vi "String to temperature device cluster.vi"(11 "Temp Device Details":string="EXCT:TYPE:UNIP:MAG:0:STAT:40000000:NICK:MB1.T1:LOOP:AUX:None:D:1.0:HTR:None:I:1.0:THTF:None:HSET:0:PIDT:OFF:ENAB:OFF:SWFL:None:FAUT:OFF:FSET:0:PIDF:None:P:1.0:SWMD:FIX:TSET:0.0000K:MAN:HVER:1:FVER:1.12:SERL:111450078:CAL:OFFS:0:COLDL:999.00K:INT:LIN:SCAL:1:FILE:None:HOTL:999.00K:TYPE:TCE:SIG:VOLT:-0.0038mV:CURR:-0.0000A:TEMP:0.0000K:POWR:0.0000W:RES:0.0000O:SLOP:0.0000O/K") -> (3 "Temperature Device Settings":T1)   [LabVIEW 2014, in "Mercury iXX.lvlib" / "Temperature.lvlib"]
uses:
  Temperature.lvlib
  Controls/Temperature Device (Read).ctl
  Controls/Manufacturing Data.ctl
  Controls/Temperature Sensor Type.ctl
  Controls/Excitation Cluster.ctl
  Controls/Excitation Type.ctl
  Controls/Calibration Cluster.ctl
  Controls/Calibration Interpolation.ctl
  Controls/Loop Cluster.ctl
  Controls/Temperature Signals Cluster.ctl
  Mercury iXX.lvlib
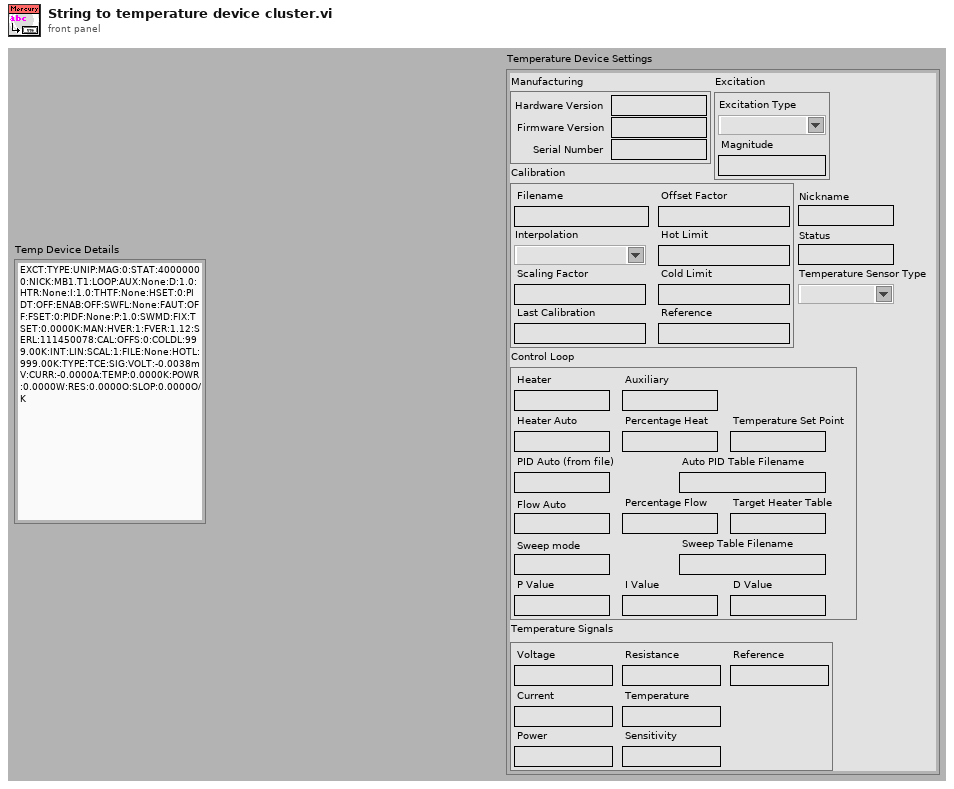
[diagram p1: front panel]
types:
  T1 = typedef "Mercury iXX.lvlib/Temperature.lvlib/Temperature Device (Read).ctl" = cluster{"Manufacturing":T2, "Temperature Sensor Type":T3, "Excitation":T4, "Calibration":T6, "Control Loop":T8, "Temperature Signals":T9, "Nickname":string, "Status":string}
  T2 = typedef "Mercury iXX.lvlib/Manufacturing Data.ctl" = cluster{"Hardware Version":string, "Firmware Version":string, "Serial Number":string}
  T3 = typedef "Mercury iXX.lvlib/Temperature.lvlib/Temperature Sensor Type.ctl" = string
  T4 = typedef "Mercury iXX.lvlib/Temperature.lvlib/Excitation Cluster.ctl" = cluster{"Excitation Type":T5, "Magnitude":string}
  T5 = typedef "Mercury iXX.lvlib/Temperature.lvlib/Excitation Type.ctl" = string
  T6 = typedef "Mercury iXX.lvlib/Temperature.lvlib/Calibration Cluster.ctl" = cluster{"Filename":string, "Interpolation":T7, "Scaling Factor":string, "Offset Factor":string, "Hot Limit":string, "Cold Limit":string, "Last Calibration":string, "Reference":string}
  T7 = typedef "Mercury iXX.lvlib/Temperature.lvlib/Calibration Interpolation.ctl" = string
  T8 = typedef "Mercury iXX.lvlib/Temperature.lvlib/Loop Cluster.ctl" = cluster{"Heater":string, "Auxiliary":string, "Heater Auto":string, "Percentage Heat":string, "Temperature Set Point":string, "PID Auto (from file)":string, "P Value":string, "I Value":string, "D Value":string, "Auto PID Table Filename":string, "Flow Auto":string, "Target Heater Table":string, "Sweep mode":string, "Sweep Table Filename":string, "Percentage Flow":string}
  T9 = typedef "Mercury iXX.lvlib/Temperature.lvlib/Temperature Signals Cluster.ctl" = cluster{"Voltage":string, "Current":string, "Power":string, "Resistance":string, "Temperature":string, "Sensitivity":string, "Reference":string}
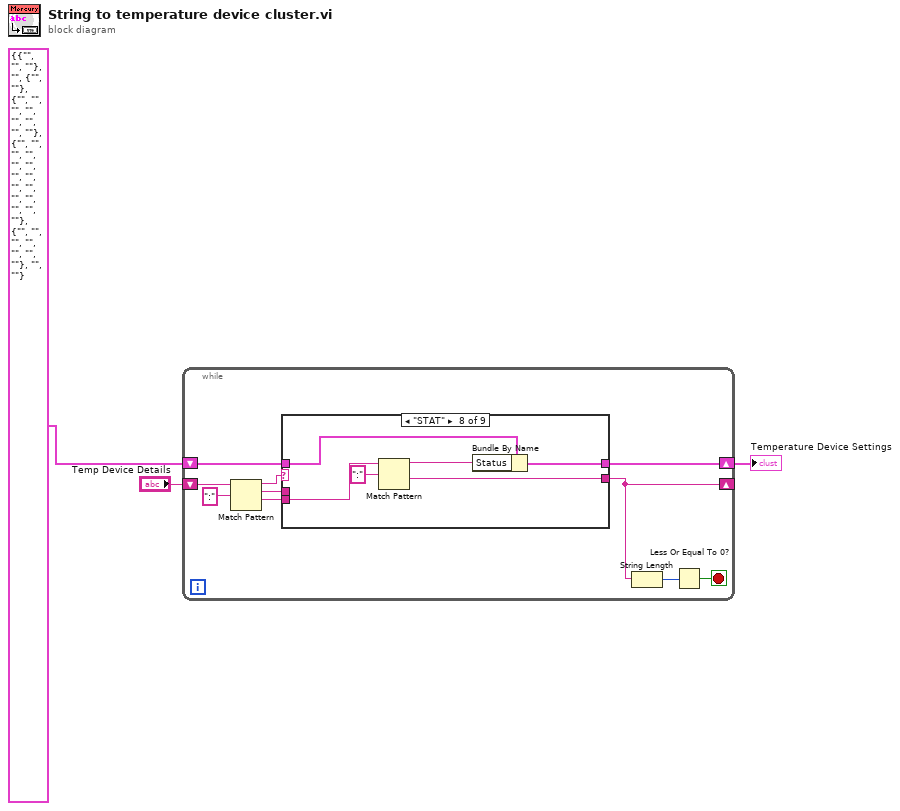
[diagram p0: block diagram]
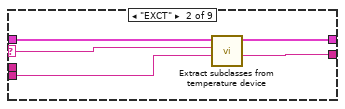
[diagram p3: hidden frame]
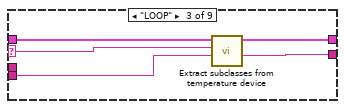
[diagram p4: hidden frame]
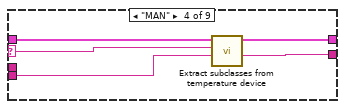
[diagram p5: hidden frame]
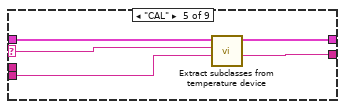
[diagram p6: hidden frame]
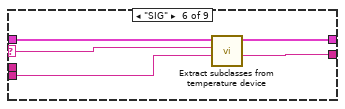
[diagram p7: hidden frame]
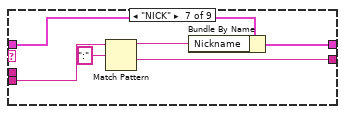
[diagram p8: hidden frame]
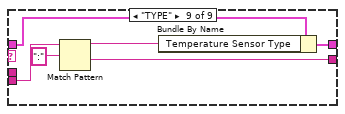
[diagram p9: hidden frame]
diagram:
  n1 = while {
    shift-right: [w8] -> w2
    shift-left: T1 {"Manufacturing"={"Hardware Version"="", "Firmware Version"="", "Serial Number"=""}, "Temperature Sensor Type"="", "Excitation"={"Excitation Type"="", "Magnitude"=""}, "Calibration"={"Filename"="", "Interpolation"="", "Scaling Factor"="", "Offset Factor"="", "Hot Limit"="", "Cold Limit"="", "Last Calibration"="", "Reference"=""}, "Control Loop"={"Heater"="", "Auxiliary"="", "Heater Auto"="", "Percentage Heat"="", "Temperature Set Point"="", "PID Auto (from file)"="", "P Value"="", "I Value"="", "D Value"="", "Auto PID Table Filename"="", "Flow Auto"="", "Target Heater Table"="", "Sweep mode"="", "Sweep Table Filename"="", "Percentage Flow"=""}, "Temperature Signals"={"Voltage"="", "Current"="", "Power"="", "Resistance"="", "Temperature"="", "Sensitivity"="", "Reference"=""}, "Nickname"="", "Status"=""} ("Temperature Device Settings 2") -> [w9]
    shift-right: [w4] -> _
    shift-left: "Temp Device Details" -> [w12]
    stop <- w10 stop-if-true
    n2 = Match Pattern(string=w12, regular expression=":") -> (before substring=w11:string, match substring=w7:string, after substring=w6:string)  [unwired: 2 out]
    n3 = case shown="\"STAT\"" w11 {
      selector: w11 -> [_ w20 w25 w30 w35 w40 _ _ _]
      tunnel: w7 -> [_ _ _ _ _ _ _ _ _]
      tunnel: w9 -> [w15 w19 w24 w29 w34 w39 w44 w50 w56]
      tunnel: [w15 w18 w23 w28 w33 w38 w43 w49 w55] -> w8
      tunnel: [w14 w17 w22 w27 w32 w37 w41 w47 w54] -> w4
      tunnel: w6 -> [w14 w16 w21 w26 w31 w36 w45 w51 w57]
      frame "", Default {
      }
      frame "EXCT" {
        n4 = call "Extract subclasses from temperature device.vi"("Data In"=w16, "Class"=w20, "Temperature Device Settings in"=w19) -> ("Data out"=w17:string, "Temperature Device Settings out"=w18:T1)  [unwired: 7 out]
      }
      frame "LOOP" {
        n5 = call "Extract subclasses from temperature device.vi"("Data In"=w21, "Class"=w25, "Temperature Device Settings in"=w24) -> ("Data out"=w22:string, "Temperature Device Settings out"=w23:T1)  [unwired: 7 out]
      }
      frame "MAN" {
        n6 = call "Extract subclasses from temperature device.vi"("Data In"=w26, "Class"=w30, "Temperature Device Settings in"=w29) -> ("Data out"=w27:string, "Temperature Device Settings out"=w28:T1)  [unwired: 7 out]
      }
      frame "CAL" {
        n7 = call "Extract subclasses from temperature device.vi"("Data In"=w31, "Class"=w35, "Temperature Device Settings in"=w34) -> ("Data out"=w32:string, "Temperature Device Settings out"=w33:T1)  [unwired: 7 out]
      }
      frame "SIG" {
        n8 = call "Extract subclasses from temperature device.vi"("Data In"=w36, "Class"=w40, "Temperature Device Settings in"=w39) -> ("Data out"=w37:string, "Temperature Device Settings out"=w38:T1)  [unwired: 7 out]
      }
      frame "NICK" {
        n9 = Match Pattern(string=w45, regular expression=":") -> (before substring=w42:string, after substring=w41:string)  [unwired: 3 out]
        n10 = Bundle By Name(cluster=w44, "Nickname"=w42) -> (w43:T1)
      }
      frame "STAT" {
        n11 = Match Pattern(string=w51, regular expression=":") -> (before substring=w48:string, after substring=w47:string)  [unwired: 3 out]
        n12 = Bundle By Name(cluster=w50, "Status"=w48) -> (w49:T1)
      }
      frame "TYPE" {
        n13 = Match Pattern(string=w57, regular expression=":") -> (before substring=w53:string, after substring=w54:string)  [unwired: 3 out]
        n14 = Bundle By Name(cluster=w56, "Temperature Sensor Type"=w53) -> (w55:T1)
      }
    }
    n15 = String Length(string=w4) -> (length=w5:i32)
    n16 = Less Or Equal To 0?(x=w5) -> (x <= 0?=w10:bool)
  }
  "Temperature Device Settings" <- w2
